vi "Voltage Collection.vi"() -> ()   [LabVIEW 2010]
panel:
  in  "stop 3":bool
  in  "stop 2":bool
  out "Gauge":dbl(knob) scale=0.0..5.0
  in  "stop":bool
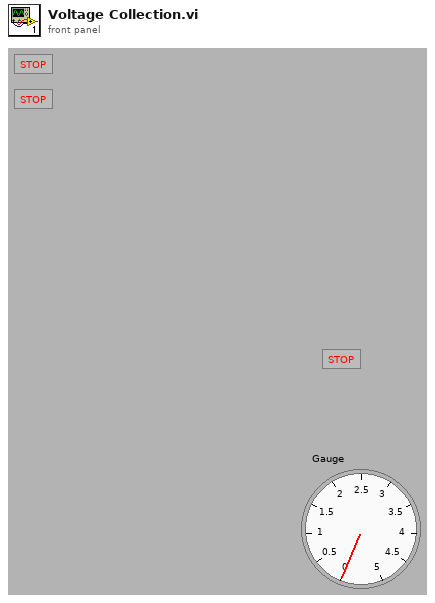
[diagram p1: front panel]
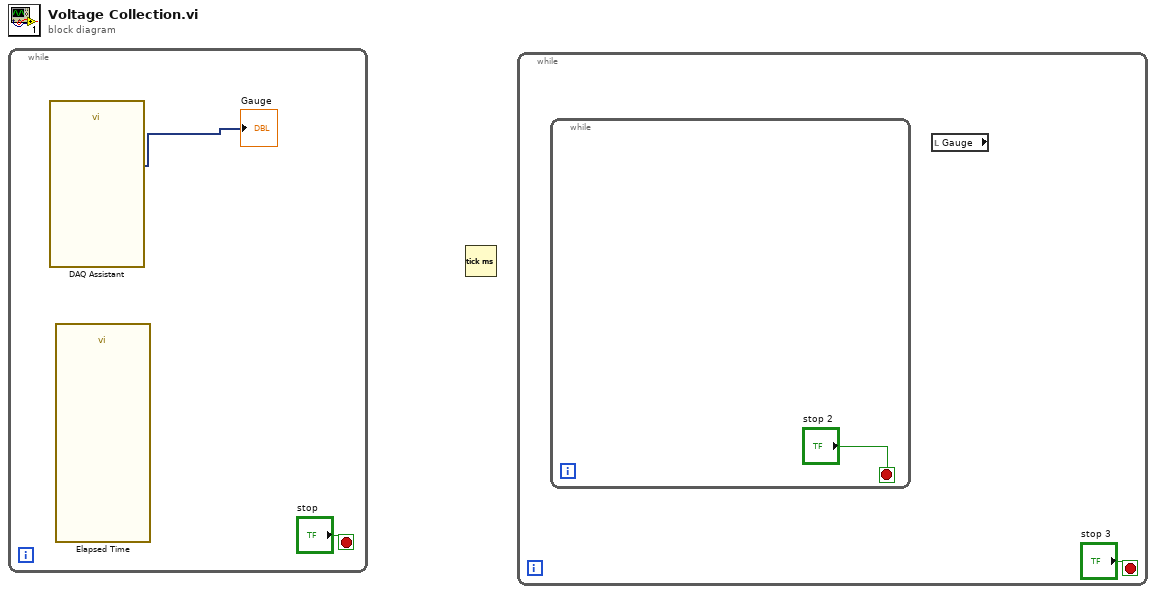
[diagram p0: block diagram]
diagram:
  n1 = while {
    stop <- "stop" stop-if-true
    n2 = call "DAQ Assistant"() -> ("data"=→"Gauge":dynamicdata)  [unwired: 17 in, 2 out]
    n3 = call "Elapsed Time"() -> ()  [unwired: 12 in, 8 out]
  }
  n4 = Tick Count (ms)() -> ()  [unwired: 1 out]
  n5 = while {
    stop <- "stop 3" stop-if-true
    n6 = while {
      stop <- "stop 2" stop-if-true
    }
    n7 = local read "Gauge"() -> ()  [unwired: 1 out]
  }
